vi "UEF Example2 Main.vi"() -> ()   [LabVIEW 2015]
uses:
  UEF Handler/UEF Handler2.lvclass
  UEF Handler/UEF Handler2.lvclass/UEF Handler2.ctl
  UEF Handler/Write RectName Ref.vi
  <vilib>/LIEF/Image Editor Handler/Image Editor Handler.lvclass
panel:
  out "error out":errorcluster
  in  "New Rectangle Name:":string
  in  "2D Picture":picture
  # "1. Run the VI and type a name in the textbox\n2. Right-click an empty space in the picture -> Add Rectangle. You can repeat (and change the textbox text).\n3. Play with the forms (double-click, move, delete...)"
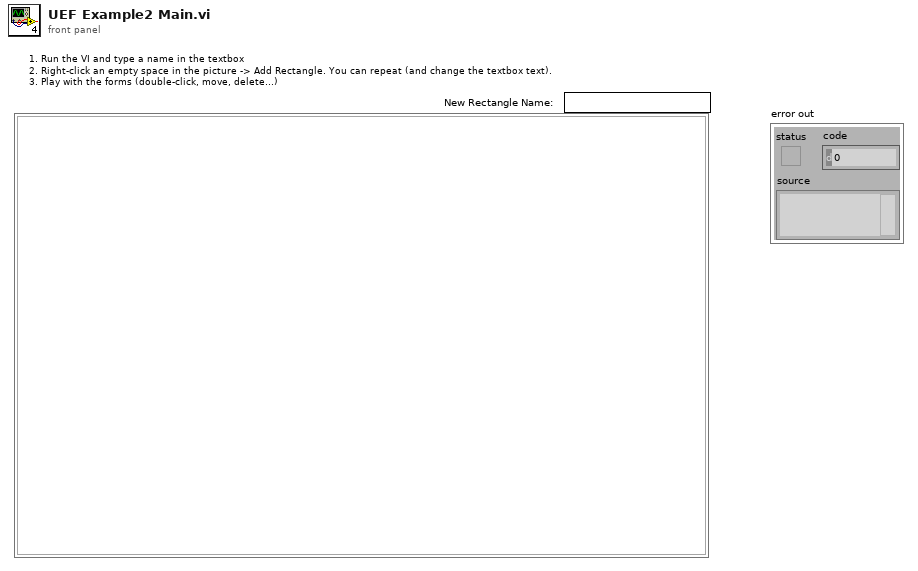
[diagram p1: front panel]
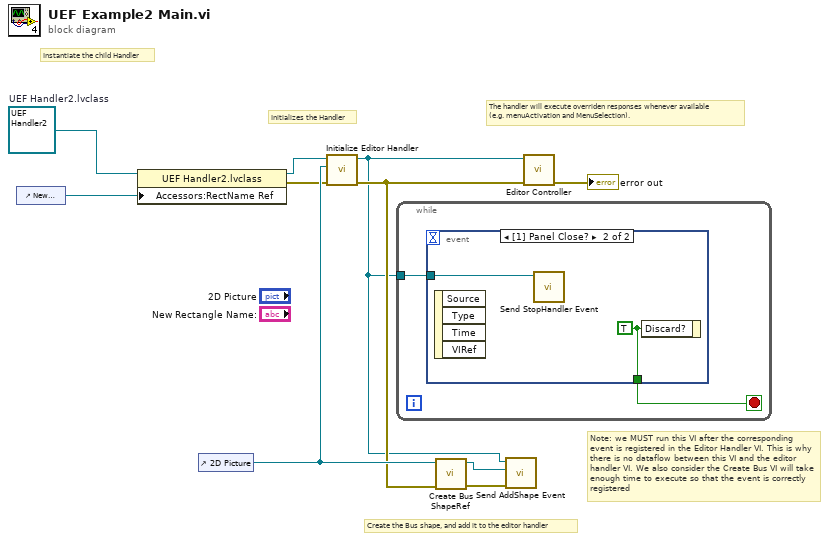
[diagram p0: block diagram]
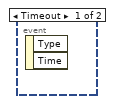
[diagram p2: hidden frame]
diagram:
  w10 = refnum<class "UEF Handler2.lvclass"> refnum  # UEF Handler2.lvclass
  # "Note: we MUST run this VI after the corresponding event is registered in the Editor Handler VI. This is why there is no dataflow between this VI and the editor handler VI. We also consider the Create Bus VI will take enough time to execute so that the event is correctly registered"
  # "Create the Bus shape, and add it to the editor handler"
  # "The handler will execute overriden responses whenever available\n(e.g. menuActivation and MenuSelection)."
  # "Initializes the Handler"
  # "Instantiate the child Handler"
  n1 = control-ref of="New Rectangle Name:"() -> (w9:refnum<vi>)
  n2 = property class="UEF Handler2.lvclass"(reference=w10, "Accessors:RectName Ref"=w9) -> (reference out=w8:refnum<class "UEF Handler2.lvclass">, error out=w1:errorcluster)  [unwired: 1 in]
  n3 = control-ref of="2D Picture"() -> (w6:refnum<vi>)
  n4 = call <vilib>:"Initialize Editor Handler.vi"("error in (no error)"=w1, "PictureRef"=w6, "Editor Handler in"=w8) -> ("error out"=w5:errorcluster, "Editor Handler out"=w4:refnum<class "UEF Handler2.lvclass">)  [unwired: 7 in]
  n5 = while {
    tunnel: w4 -> [w11]
    stop <- w12 stop-if-true
    n6 = event shown="[1] Panel Close?" {
      selector: _ -> [_ _]
      dyn-events: _ -> [_ _]
      timeout: _ -> [_ _]
      tunnel: [_ w14] -> w12
      tunnel: w11 -> [_ w13]
      event Timeout {
        n7 = event-data() -> ()  [unwired: 1 in, 2 out]
      }
      event Panel Close? {
        w14 = TRUE ("Discard?")
        n8 = event-data() -> ()  [unwired: 1 in, 4 out]
        n9 = call <vilib>:"Send StopHandler Event.vi"("Editor Handler in"=w13) -> ()  [unwired: 9 in, 2 out]
        n10 = event-data("Discard?"=w14) -> ()  [unwired: 1 in, 1 out]
      }
    }
  }
  n11 = call "Create Bus ShapeRef.vi"("error in (no error)"=w5, "Picture in"=w6) -> ("error out"=w3:errorcluster, "Data Value Reference out"=w2:refnum<data-value>)  [unwired: 8 in]
  n12 = call <vilib>:"Send AddShape Event.vi"("error in (no error)"=w3, "New Shape Reference"=w2, "Editor Handler in"=w4) -> ()  [unwired: 7 in, 2 out]
  n13 = call <vilib>:"Editor Controller.vi"("error in (no error)"=w5, "Editor Handler in"=w4) -> ("error out"=→"error out":errorcluster)  [unwired: 8 in, 1 out]
